vi "set control size.vi"(8 "error in (no error)":errorcluster, 10 "Size":T1, 11 "Ring Control in":refnum<class "Ring Control.lvclass">) -> (0 "error out":errorcluster, 3 "Ring Control out":refnum<class "Ring Control.lvclass">)   [LabVIEW 2010, in "Ring Control.lvclass"]
uses:
  Ring Control.lvclass
  <vilib>/Utility/miscctls.llb/LVBoundsTypeDef.ctl
  Ring Control.lvclass/Ring Control.ctl
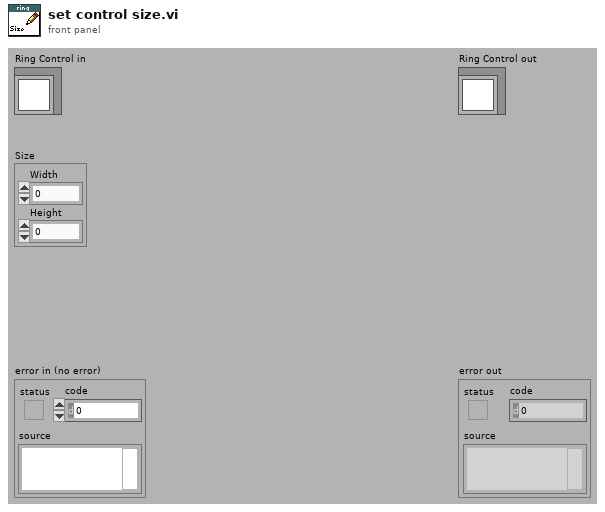
[diagram p1: front panel]
types:
  T1 = typedef "LVBoundsTypeDef.ctl" = cluster{"Width":u32, "Height":u32}
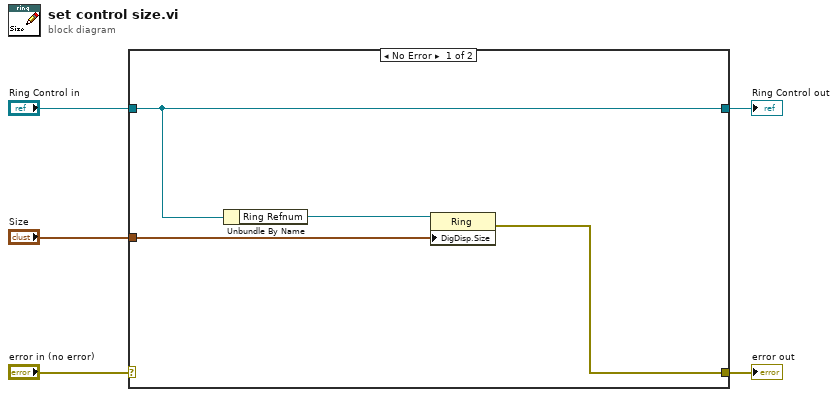
[diagram p0: block diagram]
diagram:
  n1 = case shown="No Error" "error in (no error)" {
    selector: "error in (no error)" -> [_ w11]
    tunnel: [w8 w11] -> w4
    tunnel: [w7 w10] -> w2
    tunnel: "Ring Control in" -> [w7 w10]
    tunnel: "Size" -> [w9 _]
    frame No Error {
      n2 = Unbundle By Name(w7) -> ("Ring Refnum"=w6:refnum<vi>)
      n3 = property class="Ring"(reference=w6, "DigDisp.Size"=w9) -> (error out=w8:errorcluster)  [unwired: 1 in, 1 out]
    }
    frame Error {
    }
  }
  "error out" <- w4
  "Ring Control out" <- w2
